vi "main.vi"() -> ()   [LabVIEW 2018]
panel:
  out "fault_t_pistons":bool
  out "fault_t_pneum_tank":bool
  out "fault_t_res_bat":bool
  out "fault_t_prime_bat_2":bool
  out "fault_t_prime_bat_1":bool
  in  "prim_bat_3":bool
  in  "prim_bat_2":bool
  in  "prim_bat_1":bool
  out "t_pistons":i32
  out "t_pneum_tank":i32
  out "t_res_bat":i32
  out "t_prime_bat_2":i32
  out "t_prime_bat_1":i32
  out "count_laser_l":u16
  out "count_laser_r":u16
  out "count_light_bl":u16
  out "count_light_br":u16
  out "count_light_fl":u16
  out "count_light_fr":u16
  out "voltage_3":i32
  out "voltage_2":i32
  out "voltage_1":i32
  out "current_3":i32
  out "currents_2":i32
  out "current_1":i32
  in  "solenoid_3":bool
  in  "solenoid_2":bool
  in  "solenoid_1":bool
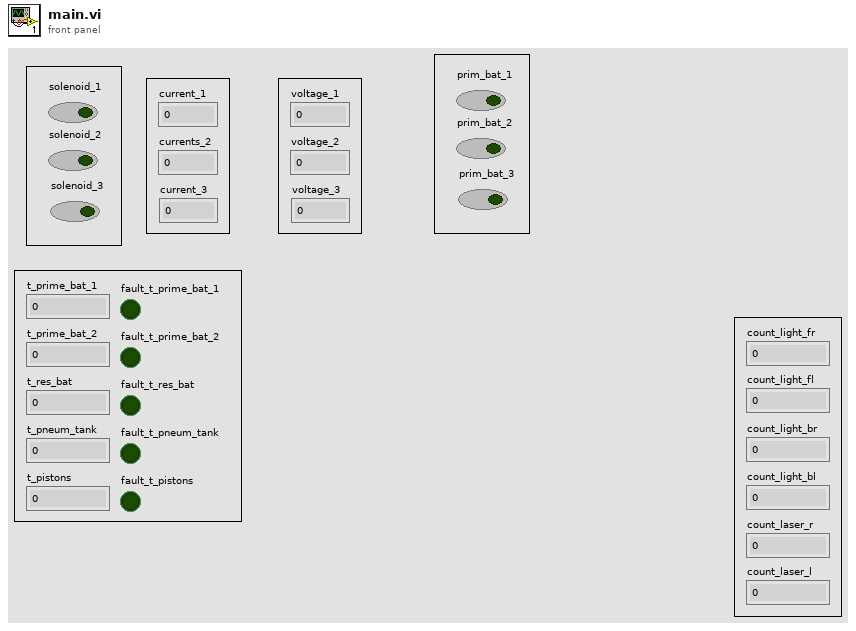
[diagram p1: front panel]
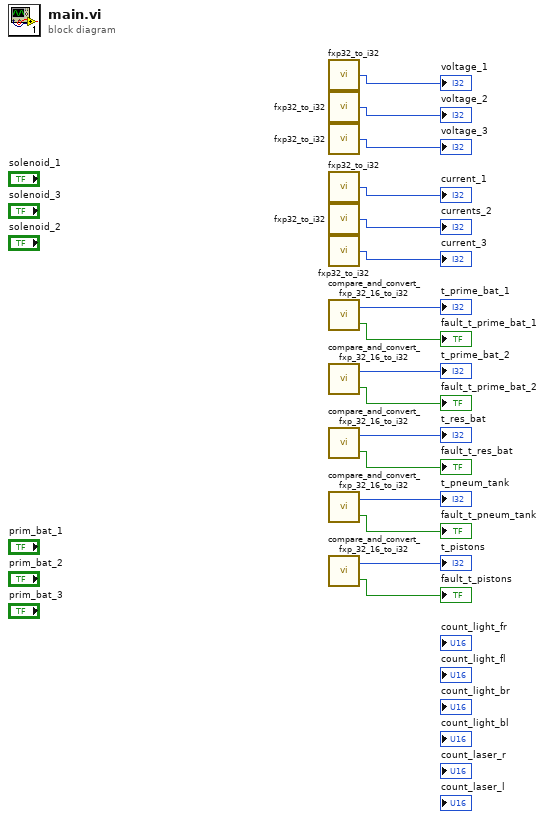
[diagram p0: block diagram]
diagram:
  n1 = call "fxp32_to_i32.vi"() -> ("32bit integer"=→"voltage_1":i32)  [unwired: 1 in]
  n2 = call "fxp32_to_i32.vi"() -> ("32bit integer"=→"voltage_2":i32)  [unwired: 1 in]
  n3 = call "fxp32_to_i32.vi"() -> ("32bit integer"=→"voltage_3":i32)  [unwired: 1 in]
  n4 = call "fxp32_to_i32.vi"() -> ("32bit integer"=→"current_1":i32)  [unwired: 1 in]
  n5 = call "fxp32_to_i32.vi"() -> ("32bit integer"=→"currents_2":i32)  [unwired: 1 in]
  n6 = call "fxp32_to_i32.vi"() -> ("32bit integer"=→"current_3":i32)  [unwired: 1 in]
  n7 = call "compare_and_convert_fxp_32_16_to_i32.vi"() -> ("out_of_range"=→"fault_t_prime_bat_1":bool, "32bit integer"=→"t_prime_bat_1":i32)  [unwired: 3 in]
  n8 = call "compare_and_convert_fxp_32_16_to_i32.vi"() -> ("out_of_range"=→"fault_t_prime_bat_2":bool, "32bit integer"=→"t_prime_bat_2":i32)  [unwired: 3 in]
  n9 = call "compare_and_convert_fxp_32_16_to_i32.vi"() -> ("out_of_range"=→"fault_t_res_bat":bool, "32bit integer"=→"t_res_bat":i32)  [unwired: 3 in]
  n10 = call "compare_and_convert_fxp_32_16_to_i32.vi"() -> ("out_of_range"=→"fault_t_pneum_tank":bool, "32bit integer"=→"t_pneum_tank":i32)  [unwired: 3 in]
  n11 = call "compare_and_convert_fxp_32_16_to_i32.vi"() -> ("out_of_range"=→"fault_t_pistons":bool, "32bit integer"=→"t_pistons":i32)  [unwired: 3 in]
